vi "CPP_AeroFlow.vi"(4 "Pressure (mBar)":dbl=1000.0, 5 "Temperature (C)":dbl=20.0, 7 "Calibration Folder Path":path=path "G:/5HoleProbe", 9 "ZeroedPressures (mmH2O)":dbl[][](array[numeric])=array820x5[4100 elements]) -> (0 "Time(ms)":u32, 1 "TotalPoints":i32, 2 "ReductionCode":i32[](array[numeric]), 3 "RawVmagUVWCone":dbl[][](array[numeric]))   [LabVIEW 2014]
uses:
  VWflipperArray.vi
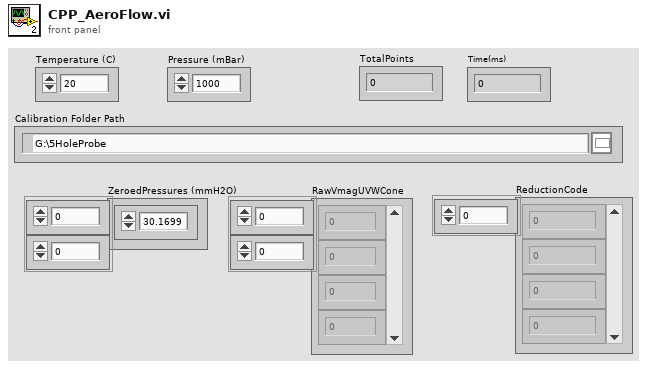
[diagram p1: front panel]
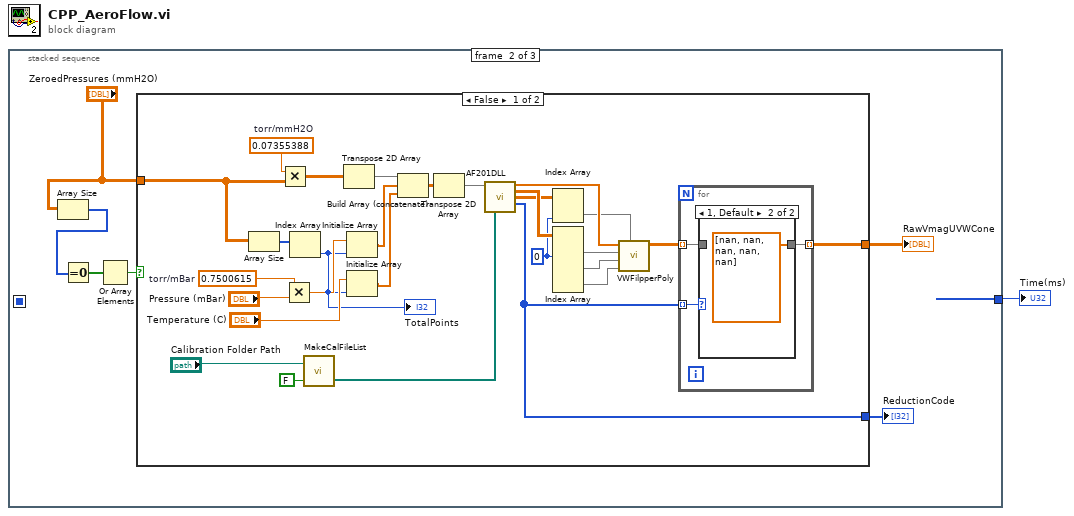
[diagram p0: block diagram]
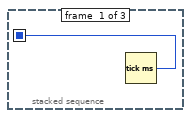
[diagram p2: hidden frame]
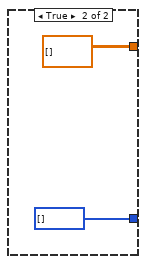
[diagram p4: hidden frame]
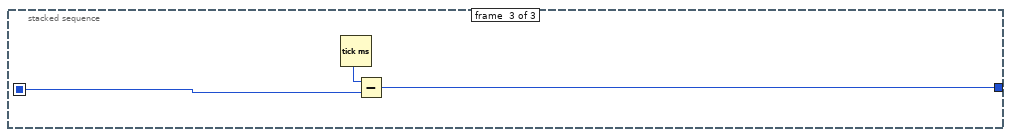
[diagram p5: hidden frame]
diagram:
  n1 = stacked-sequence {
    seq-local: [w2 _ _] -> [_ _ w44]
    tunnel: [_ _ w46] -> w1
    frame #0 {
      n2 = Tick Count (ms)() -> (millisecond timer value=w2:u32)
    }
    frame #1 {
      n3 = Array Size(array="ZeroedPressures (mmH2O)") -> (size(s)=w4:i32[])
      n4 = Equal To 0?(x=w4) -> (x = 0?=w5:bool[])
      n5 = Or Array Elements(Boolean array=w5) -> (logical OR=w3:bool)
      n6 = case shown="False" w3 {
        tunnel: "ZeroedPressures (mmH2O)" -> [w22 _]
        tunnel: [w10 dbl[][] [] ("VmagUVWCone")] -> w8
        tunnel: [w9 i32[] [] ("ErrorReduced")] -> w7
        frame False {
          w12 = 0 ("disabled index (col)")
          w34 = 0.7500615  # torr/mBar
          w14 = 0.07355388  # torr/mmH2O
          n7 = Array Size(array=w22) -> (size(s)=w19:i32[])
          n8 = Multiply(x=w14, y=w22) -> (x*y=w20:dbl[][])
          n9 = Multiply(x=w34, y="Pressure (mBar)") -> (x*y=w36:dbl)
          n10 = Index Array(array=w19) -> (element=w23:i32)  [unwired: 1 in]
          "TotalPoints" <- w23
          n11 = call "MakeCalFileList.vi"("Old5HoleProbe?"=FALSE, "Calibration Folder Path"="Calibration Folder Path") -> ("AeroFlowCals"=w28:path[])  [unwired: 1 out]
          n12 = Transpose 2D Array(2D array=w20) -> (transposed array=w15:dbl[][])
          n13 = Initialize Array(w36, w23) -> (w17:dbl[])
          n14 = Initialize Array("Temperature (C)", w23) -> (w16:dbl[])
          n15 = Build Array (concatenate)(w15, w17, w16) -> (w18:dbl[][])
          n16 = Transpose 2D Array(2D array=w18) -> (transposed array=w21:dbl[][])
          n17 = call "AF201DLL.vi"("Data to Reduce"=w21, "Calibration File(s)"=w28) -> ("Vel_Mag_calc"=w27:dbl[], "UVW_calc"=w29:dbl[][], "angles_calc(Cone/Roll/Alpha/Beta)"=w25:dbl[][], "ErrorReduced"=w9:i32[])  [unwired: 10 in]
          n18 = Index Array(array=w25, index (col)=w12) -> (element=w26:dbl[])  [unwired: 1 in]
          n19 = Index Array(array=w29, index (col) #1=w12) -> (element #1=w30:dbl[], element #2=w31:dbl[], element #3=w32:dbl[])  [unwired: 5 in]
          n20 = call-poly "VWFilpperPoly.vi"("Theta Degree"=w26, "Probe w m/s"=w32, "Probe v m/s"=w31, "Probe u  m/s"=w30, "VMagn m/s"=w27) -> ("VmagUVWCone"=w11:dbl[][])  [unwired: 6 in]
          n21 = for {
            tunnel: w11 -> [w37] mode=indexing
            tunnel: w9 -> [w39] mode=indexing
            tunnel: [w38] -> w10 mode=indexing
            n22 = case shown="1, Default" w39 {
              tunnel: [w40 dbl[] [nan, nan, nan, nan, nan] ("VmagUVWCone")] -> w38
              tunnel: w37 -> [w40 _]
              frame 0 {
              }
              frame 1, Default {
              }
            }
          }
        }
        frame True {
        }
      }
      "RawVmagUVWCone" <- w8
      "ReductionCode" <- w7
    }
    frame #2 {
      n23 = Tick Count (ms)() -> (millisecond timer value=w45:u32)
      n24 = Subtract(x=w45, y=w44) -> (x-y=w46:u32)
    }
  }
  "Time(ms)" <- w1
